vi "Default Values.vi"() -> ()   [LabVIEW 2012, in "Waveform Data Logger Shared.lvlib"]
uses:
  Waveform Data Logger Shared.lvlib
panel:
  in  "Q Size":i32=5
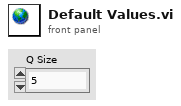
[diagram p1: front panel]
diagram:
